vi "take_data (SubVI).vi"(7 "trig?":bool, 8 "instrum in":T1, 11 "channel settings":T3={"samples per channel"=1000, "sampling rate"=1000.0, "data task"="", "drive channel"="", "Clock src"="", "synth trigger"=""} {"sampling rate" format="%0.2f"}) -> (0 "instrum out":T1, 2 "data tasks":T2, 3 "Actual Sample Rate":dbl=10000.0 format="%0.2f")   [LabVIEW 2014]
uses:
  <vilib>/DAQmx/create/channels.llb/DAQmx Create Channel (AO-Voltage-Basic).vi
  <vilib>/DAQmx/configure/timing.llb/DAQmx Timing (Sample Clock).vi
  <vilib>/DAQmx/create/channels.llb/DAQmx Create Channel (AI-Voltage-Basic).vi
  <vilib>/DAQmx/configure/trigger.llb/DAQmx Start Trigger (Digital Edge).vi
  <vilib>/DAQmx/write.llb/DAQmx Write (Analog 1D DBL 1Chan NSamp).vi
  <resource>/objmgr/daqmx.rc
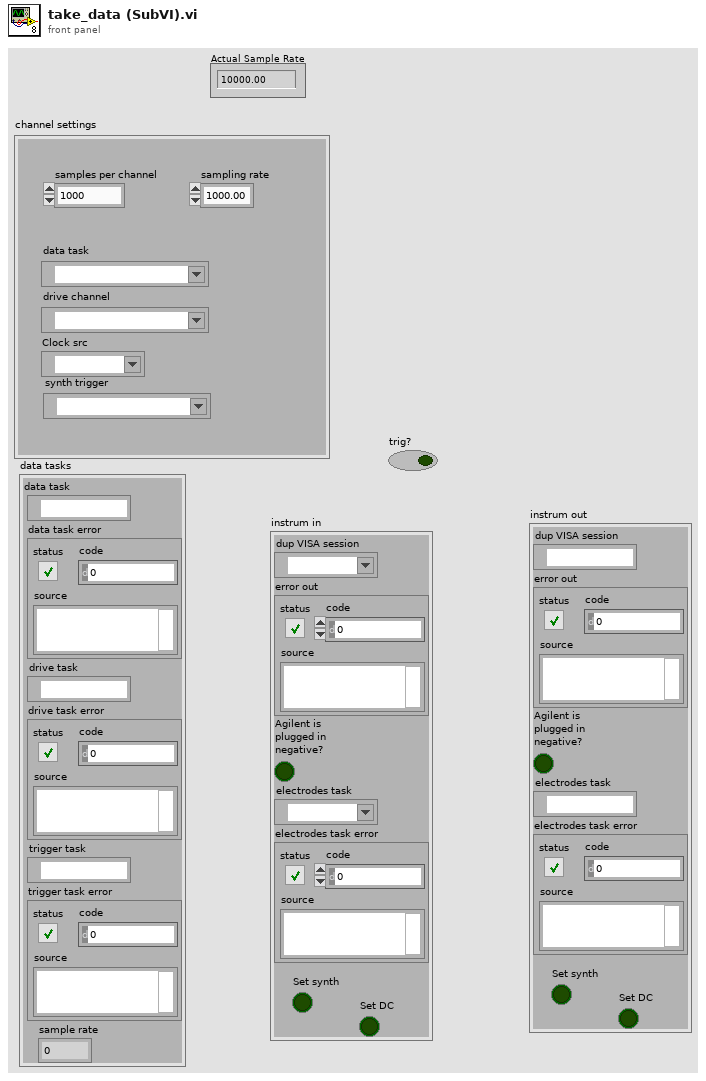
[diagram p1: front panel]
types:
  T1 = cluster{"dup VISA session":refnum<visa-resource-name>, "error out":errorcluster, "Agilent is \nplugged in \nnegative?":bool, "electrodes task":refnum<k21>, "electrodes task error":errorcluster, "Set synth":bool, "Set DC":bool}
  T2 = cluster{"data task":refnum<k21>, "data task error":errorcluster, "drive task":refnum<k21>, "drive task error":errorcluster, "trigger task":refnum<k21>, "trigger task error":errorcluster, "sample rate":dbl}
  T3 = cluster{"samples per channel":i32, "sampling rate":dbl, "data task":tag, "drive channel":tag, "Clock src":tag, "synth trigger":tag}
  T4 = cluster{"task out":refnum<k21>, "error out":errorcluster, "task out":refnum<k21>, "error out":errorcluster, "task out":refnum<k21>, "error out":errorcluster, "SampClk.Rate":dbl}
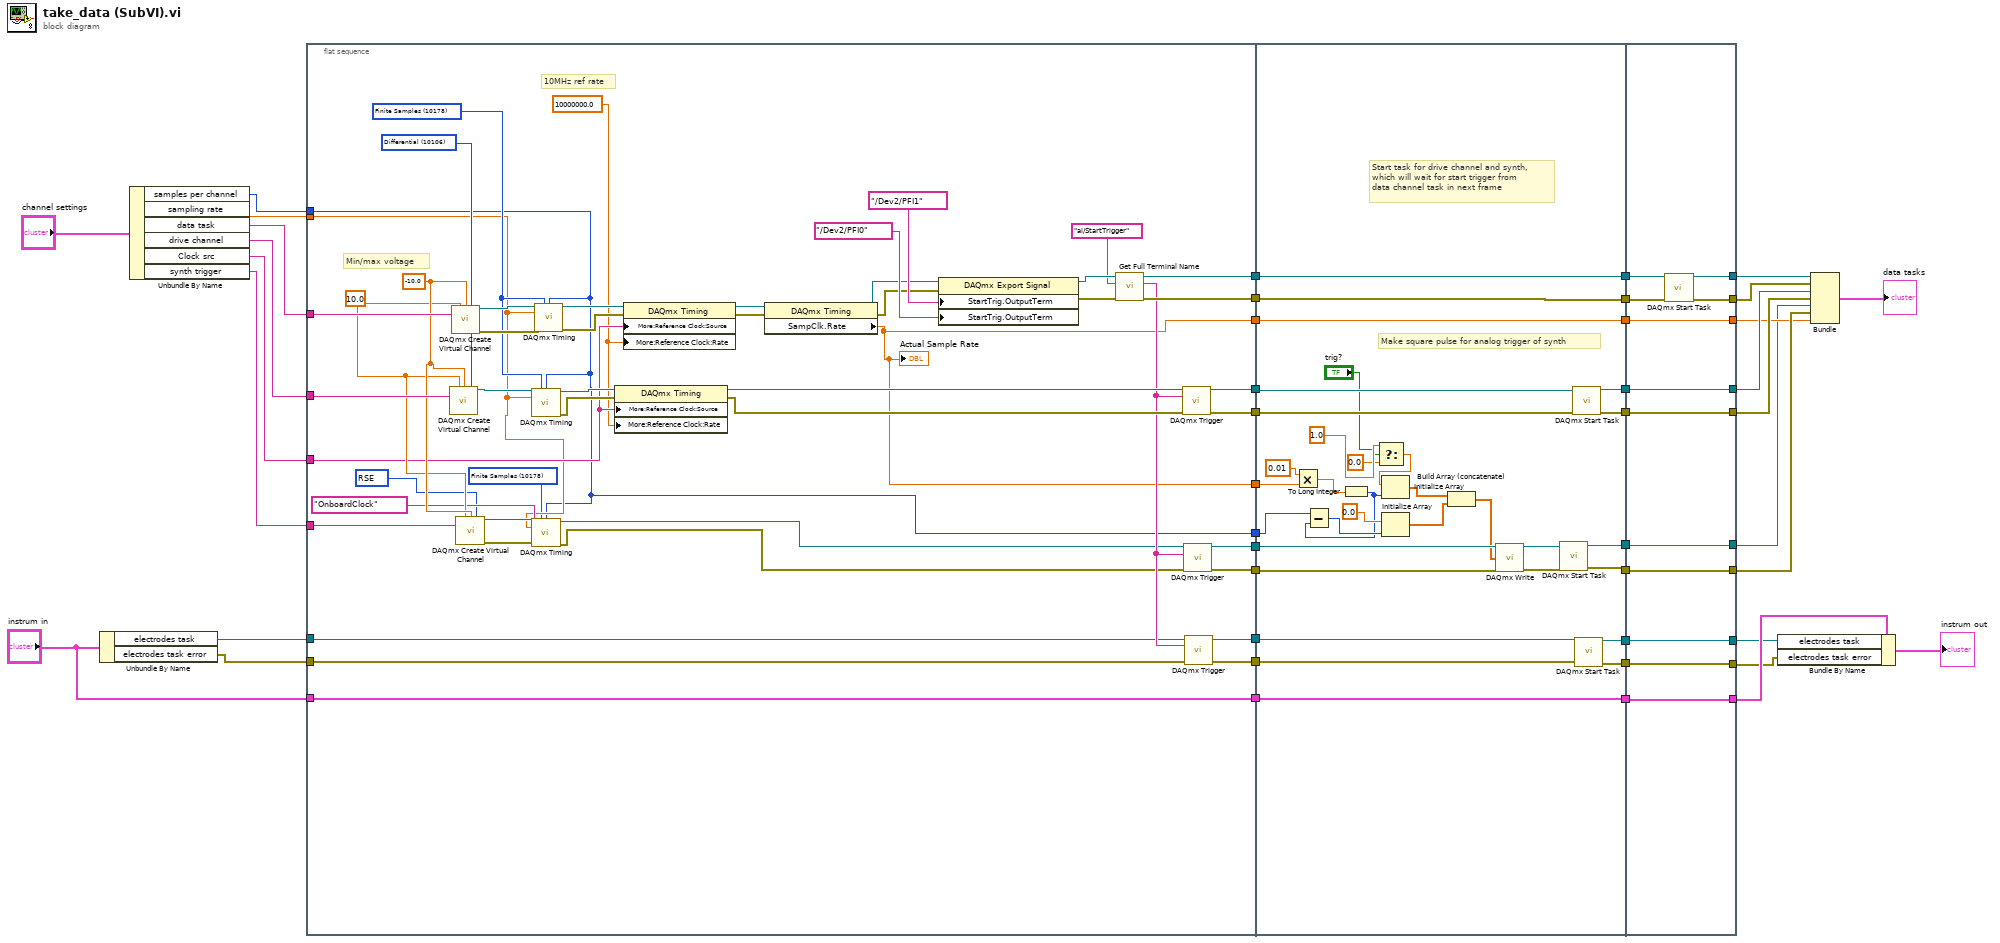
[diagram p0: block diagram]
diagram:
  n1 = Unbundle By Name("instrum in") -> ("electrodes task"=w17:refnum<k21>, "electrodes task error"=w16:errorcluster)
  n2 = Unbundle By Name("channel settings") -> ("samples per channel"=w38:i32, "sampling rate"=w40:dbl, "data task"=w43:tag, "drive channel"=w42:tag, "Clock src"=w39:tag, "synth trigger"=w41:tag)
  n3 = flat-sequence {
    tunnel: w43 -> [w72]
    tunnel: w42 -> [w71]
    tunnel: w41 -> [w70]
    tunnel: w40 -> [w49]
    tunnel: w39 -> [w54]
    tunnel: w38 -> [w45]
    tunnel: [w69] -> w37
    tunnel: [w68] -> w36
    tunnel: [w67] -> w35
    tunnel: [w66] -> w34
    tunnel: [w65] -> w33
    tunnel: [w64] -> w32
    tunnel: [w46] -> w21
    tunnel: w17 -> [w58]
    tunnel: w16 -> [w62]
    tunnel: [w61] -> w15
    tunnel: [w60] -> w14
    tunnel: "instrum in" -> [w59]
    tunnel: [w59] -> w11
    tunnel: [w45] -> w2
    tunnel: [w46] -> w1
    tunnel: w37 -> [w125]
    tunnel: w36 -> [w124]
    tunnel: w35 -> [w123]
    tunnel: w34 -> [w122]
    tunnel: w33 -> [w113]
    tunnel: w32 -> [w112]
    tunnel: [w125] -> w31
    tunnel: [w124] -> w30
    tunnel: [w121] -> w29
    tunnel: [w120] -> w28
    tunnel: [w109] -> w27
    tunnel: w21 -> [w119]
    tunnel: [w119] -> w19
    tunnel: w15 -> [w118]
    tunnel: w14 -> [w117]
    tunnel: [w116] -> w12
    tunnel: w11 -> [w116]
    tunnel: [w115] -> w7
    tunnel: [w114] -> w6
    tunnel: [w108] -> w3
    tunnel: w2 -> [w104]
    tunnel: w1 -> [w102]
    tunnel: w31 -> [w137]
    tunnel: w30 -> [w136]
    tunnel: w29 -> [w135]
    tunnel: w28 -> [w134]
    tunnel: [w135] -> w22
    tunnel: [w134] -> w23
    tunnel: [w133] -> w26
    tunnel: [w132] -> w25
    tunnel: w27 -> [w131]
    tunnel: [w131] -> w24
    tunnel: [w130] -> w20
    tunnel: w19 -> [w130]
    tunnel: w12 -> [w129]
    tunnel: [w129] -> w10
    tunnel: [w128] -> w8
    tunnel: w7 -> [w128]
    tunnel: w6 -> [w127]
    tunnel: [w127] -> w5
    tunnel: [w126] -> w4
    tunnel: w3 -> [w126]
    frame #0 {
      w48 = 10083 items=["Default"=-1, "RSE"=10083, "Differential"=10106, "Pseudodifferential"=12529] ("output terminal configuration")
      w47 = 10178 items=["Finite Samples"=10178, "Continuous Samples"=10123, "Hardware Timed Single Point"=12522] ("sample mode")
      w57 = -10.0 ("minimum value")
      w56 = 10.0 ("maximum value")
      w73 = 10106 items=["default"=-1, "RSE"=10083, "NRSE"=10078, "Differential"=10106, "Pseudodifferential"=12529] ("input terminal configuration")
      w55 = 10178 items=["Finite Samples"=10178, "Continuous Samples"=10123, "Hardware Timed Single Point"=12522] ("sample mode")
      w53 = 10000000.0 ("RefClk.Rate")
      # "10MHz ref rate"
      # "Min/max voltage"
      n4 = call-poly <vilib>:"DAQmx Create Virtual Channel.vi"("maximum value"=w56, "minimum value"=w57, "input terminal configuration"=w73, "physical channels"=w71) -> ("task out"=w76:refnum<k21>)  [unwired: 10 in, 1 out]
      n5 = call-poly <vilib>:"DAQmx Create Virtual Channel.vi"("maximum value"=w56, "minimum value"=w57, "input terminal configuration"=w73, "physical channels"=w72) -> ("task out"=w74:refnum<k21>, "error out"=w75:errorcluster)  [unwired: 10 in]
      n6 = call-poly <vilib>:"DAQmx Create Virtual Channel.vi"("maximum value"=w56, "minimum value"=w57, "output terminal configuration"=w48, "physical channels"=w70) -> ("task out"=w92:refnum<k21>, "error out"=w93:errorcluster)  [unwired: 10 in]
      n7 = call-poly <vilib>:"DAQmx Timing.vi"("task/channels in"=w76, "sample mode"=w55, "samples per channel"=w45, "rate"=w49) -> ("task out"=w79:refnum<k21>, "error out"=w80:errorcluster)  [unwired: 10 in]
      n8 = call-poly <vilib>:"DAQmx Timing.vi"("task/channels in"=w92, "sample mode"=w47, "samples per channel"=w45, "rate"=w49, "source"=tag "OnboardClock", "error in"=w93) -> ("task out"=w52:refnum<k21>, "error out"=w51:errorcluster)  [unwired: 8 in]
      n9 = call-poly <vilib>:"DAQmx Timing.vi"("task/channels in"=w74, "sample mode"=w55, "samples per channel"=w45, "rate"=w49, "error in"=w75) -> ("task out"=w77:refnum<k21>, "error out"=w78:errorcluster)  [unwired: 9 in]
      n10 = property class="DAQmx Timing"(reference=w79, error in=w80, "More:Reference Clock:Source"=w54, "More:Reference Clock:Rate"=w53) -> (reference out=w84:refnum<k21>, error out=w85:errorcluster)
      n11 = property class="DAQmx Timing"(reference=w77, error in=w78, "More:Reference Clock:Source"=w54, "More:Reference Clock:Rate"=w53) -> (reference out=w81:refnum<k21>, error out=w82:errorcluster)
      n12 = property class="DAQmx Timing"(reference=w81, error in=w82) -> (reference out=w86:refnum<k21>, error out=w88:errorcluster, "SampClk.Rate"=w46:dbl)
      "Actual Sample Rate" <- w46
      n13 = property class="DAQmx Export Signal"(reference=w86, error in=w88, "StartTrig.OutputTerm"=tag "/Dev2/PFI1", "StartTrig.OutputTerm"=tag "/Dev2/PFI0" ("10MHzRefClk.OutputTerm")) -> (reference out=w87:refnum<k21>, error out=w89:errorcluster)
      n14 = call "Get Full Terminal Name.vi"("error in (no error)"=w89, "Local Terminal Name"="ai/StartTrigger", "task/channels in"=w87) -> ("error out"=w68:errorcluster, "Terminal Name with Device Prefix"=w63:tag, "task out"=w69:refnum<k21>)  [unwired: 6 in]
      n15 = call-poly <vilib>:"DAQmx Trigger.vi"("task/channels in"=w84, "source"=w63, "error in"=w85) -> ("task out"=w67:refnum<k21>, "error out"=w66:errorcluster)  [unwired: 11 in]
      n16 = call-poly <vilib>:"DAQmx Trigger.vi"("task/channels in"=w52, "source"=w63, "error in"=w51) -> ("task out"=w65:refnum<k21>, "error out"=w64:errorcluster)  [unwired: 11 in]
      n17 = call-poly <vilib>:"DAQmx Trigger.vi"("task/channels in"=w58, "source"=w63, "error in"=w62) -> ("task out"=w61:refnum<k21>, "error out"=w60:errorcluster)  [unwired: 11 in]
    }
    frame #1 {
      # "Start task for drive channel and synth,\nwhich will wait for start trigger from \ndata channel task in next frame"
      # "Make square pulse for analog trigger of synth"
      n18 = Multiply(x=0.01, y=w102) -> (x*y=w100:dbl)
      n19 = To Long Integer(number=w100) -> (32bit integer=w99:i32)
      n20 = Subtract(x=w104, y=w99) -> (x-y=w103:i32)
      n21 = Select(t=1.0 ("element"), s="trig?", f=0.0) -> (s? t:f=w96:dbl)
      n22 = Initialize Array(w96, w99) -> (w106:dbl[])
      n23 = Initialize Array(0.0 ("element"), w103) -> (w105:dbl[])
      n24 = Build Array (concatenate)(w106, w105) -> (w98:dbl[])
      n25 = call-poly <vilib>:"DAQmx Write.vi"("task/channels in"=w113, "data"=w98, "error in"=w112) -> ("task out"=w111:refnum<k21>, "error out"=w110:errorcluster)  [unwired: 10 in, 1 out]
      n26 = call <vilib>:"DAQmx Start Task.vi"("task/channels in"=w111, "error in"=w110) -> ("task out"=w108:refnum<k21>, "error out"=w109:errorcluster)  [unwired: 12 in]
      n27 = call <vilib>:"DAQmx Start Task.vi"("task/channels in"=w123, "error in"=w122) -> ("task out"=w121:refnum<k21>, "error out"=w120:errorcluster)  [unwired: 12 in]
      n28 = call <vilib>:"DAQmx Start Task.vi"("task/channels in"=w118, "error in"=w117) -> ("task out"=w115:refnum<k21>, "error out"=w114:errorcluster)  [unwired: 12 in]
    }
    frame #2 {
      n29 = call <vilib>:"DAQmx Start Task.vi"("task/channels in"=w137, "error in"=w136) -> ("task out"=w133:refnum<k21>, "error out"=w132:errorcluster)  [unwired: 12 in]
    }
  }
  n30 = Bundle By Name(cluster=w10, "electrodes task"=w8, "electrodes task error"=w5) -> (→"instrum out":T1)
  n31 = Bundle("task out"=w26, "error out"=w25, "task out"=w22, "error out"=w23, "task out"=w4, "error out"=w24, "SampClk.Rate"=w20) -> (→"data tasks":T4)  [unwired: 1 in]
